vi "Yokogawa WT1800 Series Measure Integrate.vi"() -> ()   [LabVIEW 2015]
doc: "This example shows how to measure the integrate data."
uses:
  <instrlib>/Yokogawa WT1800 Series/Public/Utility/Function/Create Function String (Integrate).vi
  <instrlib>/Yokogawa WT1800 Series/Public/Data/Low Level/Fetch Measurement (Normal).vi
  <instrlib>/Yokogawa WT1800 Series/Yokogawa WT1800 Series.lvlib
panel:
  out "Function":string[](array[string])
  out "Measurement":dbl[](array[numeric])
  in  "stop":bool
  in  "Update Rate (500ms)":dbl(ring)=0.5 items=["50m"=0.05, "100m"=0.1, "200m"=0.2, "500m"=0.5, "1"=1.0, "2"=2.0, "5"=5.0, "10"=10.0, "20"=20.0]
  in  "Element/Wiring Unit (1: 1)":i32(ring)=1 items=["1"=1, "2"=2, "3"=3, "4"=4, "5"=5, "6"=6, "Sigma A"=7, "Sigma B"=8, "Sigma C"=9]
  in  "Timeout (10000 ms)":i32=10000 min=1
  in  "VISA resource name":refnum<visa-resource-name>
  # "(c) 2011 Yokogawa Meters & Instruments Corporation.  All rights reserved."
  # "WT1800 SERIES POWER ANALYZER"
  # "s"
  # "ms"
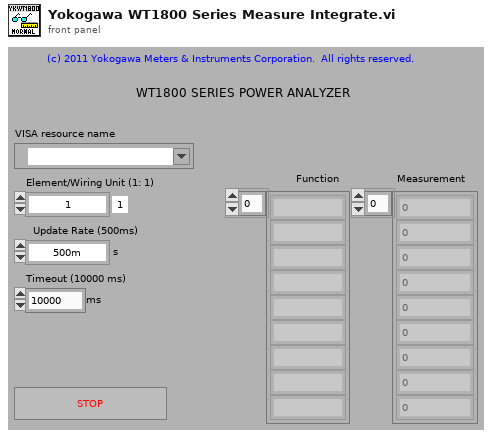
[diagram p1: front panel]
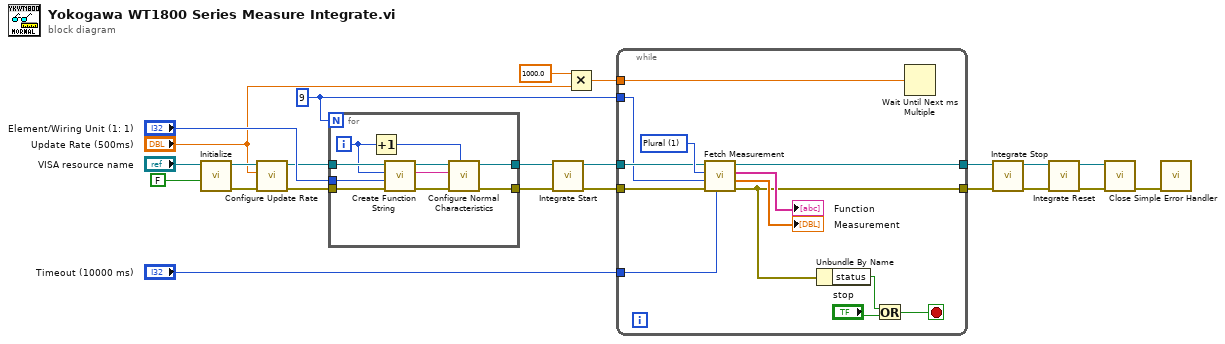
[diagram p0: block diagram]
diagram:
  w14 = 9
  n1 = call <instrlib>:"Initialize.vi"("Reset (True)"=FALSE ("Reset? (True)"), "VISA resource name"="VISA resource name") -> ("error out"=w16:errorcluster, "VISA resource name out"=w18:refnum<visa-resource-name>)  [unwired: 8 in]
  n2 = call <instrlib>:"Configure Update Rate.vi"("error in (no error)"=w16, "Update Rate (500m s)"="Update Rate (500ms)", "VISA resource name"=w18) -> ("error out"=w15:errorcluster, "VISA resource name out"=w17:refnum<visa-resource-name>)  [unwired: 7 in]
  n3 = for {
    N: w14 -> [_]
    tunnel: [w33] -> w2
    tunnel: [w32] -> w1
    tunnel: "Element/Wiring Unit (1: 1)" -> [w28]
    tunnel: w17 -> [w27]
    tunnel: w15 -> [w26]
    i -> [w25]
    n4 = Increment(x=w25) -> (x+1=w24:i32)
    n5 = call-poly <instrlib>:"Create Function String.vi"("error in (no error)"=w26, "Element/Wiring Unit (1: 1)"=w28, "Function (0: Time)"=w25, "VISA resource name"=w27) -> ("error out"=w29:errorcluster, "Function String"=w31:string, "VISA resource name out"=w30:refnum<visa-resource-name>)  [unwired: 5 in]
    n6 = call <instrlib>:"Configure Normal Characteristics.vi"("Item (1)"=w24, "error in (no error)"=w29, "Function (Empty)"=w31, "VISA resource name"=w30) -> ("error out"=w32:errorcluster, "VISA resource name out"=w33:refnum<visa-resource-name>)  [unwired: 6 in]
  }
  n7 = call <instrlib>:"Integrate Start.vi"("error in (no error)"=w1, "VISA resource name"=w2) -> ("error out"=w12:errorcluster, "VISA resource name out"=w13:refnum<visa-resource-name>)  [unwired: 8 in]
  n8 = Multiply(x=1000.0, y="Update Rate (500ms)") -> (x*y=w8:dbl)
  n9 = while {
    tunnel: [w35] -> w11
    tunnel: [w34] -> w10
    tunnel: "Timeout (10000 ms)" -> [w46]
    tunnel: w13 -> [w44]
    tunnel: w12 -> [w43]
    tunnel: w14 -> [w42]
    tunnel: w8 -> [w36]
    stop <- w39 stop-if-true
    w45 = 1 items=["One", "Plural"] ("Measure Item (1: Plural)")
    n10 = call-poly <instrlib>:"Fetch Measurement.vi"("Timeout (10000 ms)"=w46, "error in (no error)"=w43, "Number of Item (15)"=w42, "Measure Item (1: Plural)"=w45, "VISA resource name"=w44) -> ("error out"=w34:errorcluster, "Measurement"=→"Measurement":dbl[], "Function"=→"Function":string[], "VISA resource name out"=w35:refnum<visa-resource-name>)  [unwired: 3 in]
    n11 = Unbundle By Name ("名前でバンドル解除")(w34) -> ("status"=w40:bool)
    n12 = Or(x=w40, y="stop") -> (x .or. y?=w39:bool)
    n13 = Wait Until Next ms Multiple(millisecond multiple=w36) -> ()  [unwired: 1 out]
  }
  n14 = call <instrlib>:"Integrate Stop.vi"("error in (no error)"=w10, "VISA resource name"=w11) -> ("error out"=w4:errorcluster, "VISA resource name out"=w6:refnum<visa-resource-name>)  [unwired: 8 in]
  n15 = call <instrlib>:"Integrate Reset.vi"("error in (no error)"=w4, "VISA resource name"=w6) -> ("error out"=w3:errorcluster, "VISA resource name out"=w5:refnum<visa-resource-name>)  [unwired: 8 in]
  n16 = call <instrlib>:"Close.vi"("error in (no error)"=w3, "VISA resource name"=w5) -> ("error out"=w23:errorcluster)  [unwired: 9 in]
  n17 = call <vilib>:"Simple Error Handler.vi"("error in (no error)"=w23) -> ()  [unwired: 4 in, 5 out]
